vi "Parse File.vi"(8 "error in":errorcluster, 11 "File name":path=path "C:/Data/April_2019/042419/sp0006_042419.tdms") -> (0 "error out":errorcluster, 1 "Dir 2":string, 2 "Dir 1":string, 3 "<JSON>":string, 4 "metadata":string, 5 "File name":string, 6 "Lab notebook entry":string, 7 "Date time":timestamp)   [LabVIEW 2020]
uses:
  55103850-15ef-4a18-9388-7b0eadcdd449.vi
  <vilib>/JDP Science/JSONtext/Variant to JSON Text.vi
panel:
  in  "OSF Project":T1={"data"={"type"="nodes", "attributes"={"title"="", "description"="", "public"=FALSE, "category"=""}}}
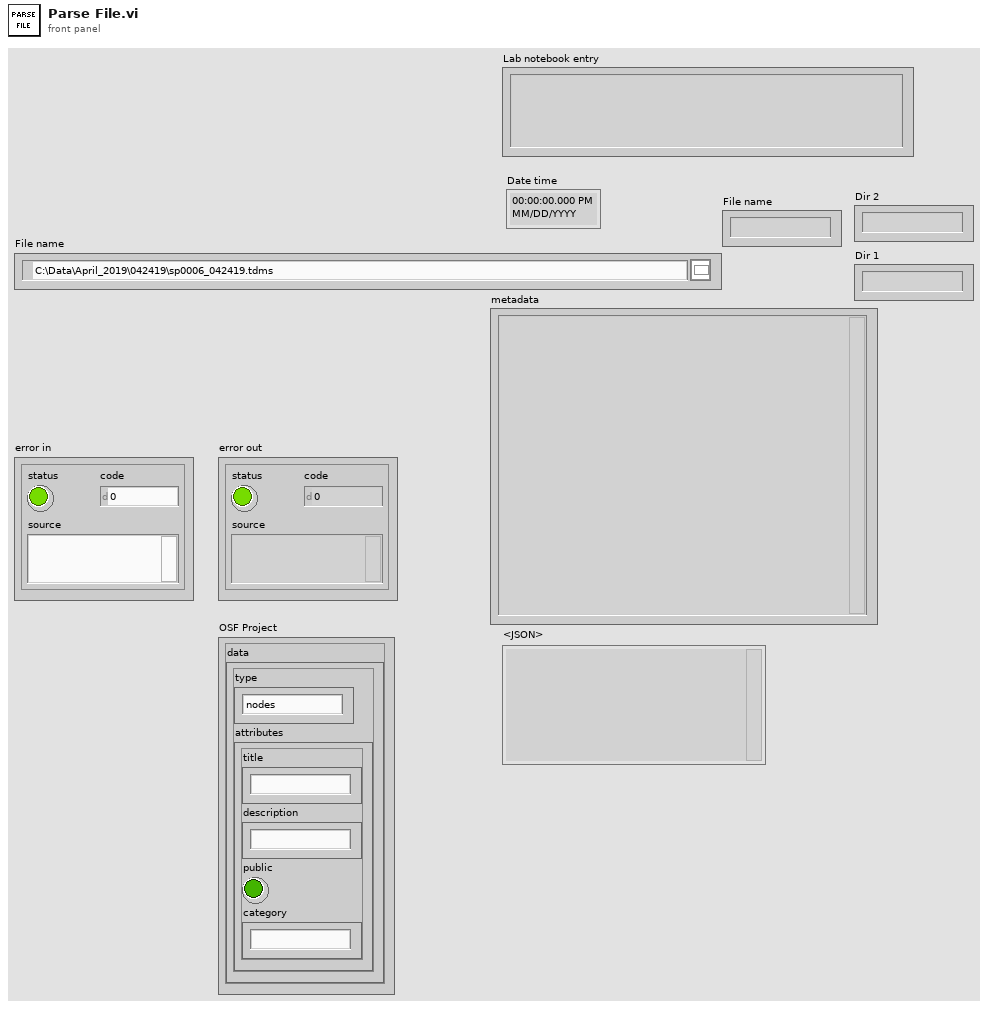
[diagram p1: front panel]
types:
  T1 = cluster{"data":cluster{"type":string, "attributes":cluster{"title":string, "description":string, "public":bool, "category":string}}}
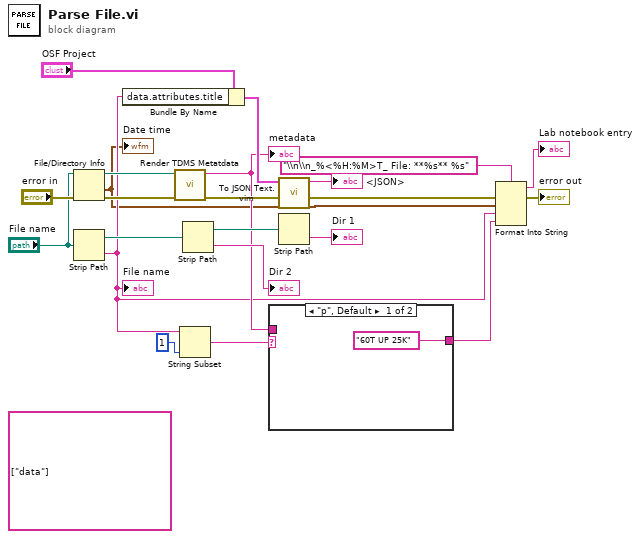
[diagram p0: block diagram]
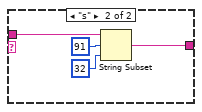
[diagram p2: hidden frame]
diagram:
  (unwired) string[] ["data"] ("Item Names")
  n1 = File/Directory Info(path="File name", error in="error in") -> (path out=w11:path, last mod=w1:timestamp, error out=w13:errorcluster)  [unwired: 4 out]
  "Date time" <- w1
  n2 = Strip Path(path="File name") -> (stripped path=w19:path, name=w2:string)
  "File name" <- w2
  n3 = Bundle By Name(cluster="OSF Project", "data.attributes.title"=w2) -> (w21:T1)
  n4 = call "Render TDMS Metatdata.vi"("error in"=w13, "File Path"=w11) -> ("error out"=w15:errorcluster, "Rendered metadata"=w5:string)  [unwired: 7 in, 1 out]
  "metadata" <- w5
  n5 = String Subset(string=w2, length (rest)=1 ("length (rest)")) -> (substring=w3:string)  [unwired: 1 in]
  n6 = Strip Path(path=w19) -> (stripped path=w17:path, name=→"Dir 2":string)
  n7 = case shown="\"p\", Default" w3 {
    tunnel: ["60T UP 25K" ("Rendered metadata") w25] -> w9
    tunnel: w5 -> [_ w24]
    frame "p", Default {
    }
    frame "s" {
      n8 = String Subset(string=w24, offset (0)=91, length (rest)=32 ("length (rest)")) -> (substring=w25:string)
    }
  }
  n9 = call "To JSON Text.vim"("error in (no error)"=w15, "Anything"=w21) -> ("error out"=w8:errorcluster, "<JSON>"=→"<JSON>":string)  [unwired: 8 in]
  n10 = Strip Path(path=w17) -> (name=→"Dir 1":string)  [unwired: 1 out]
  n11 = Format Into String(format string="\\n\\n_%<%H:%M>T_ File: **%s** %s", error in=w8, w1, w2, w9) -> (resulting string=→"Lab notebook entry":string, error out=→"error out":errorcluster)  [unwired: 1 in]
